vi "Destory for traverse.vi"(8 "error in (no error)":errorcluster caption="错误输入（无错误）", 11 "Class in":refnum<class "PanelRootNode.lvclass"> caption="DNL_LabVIEW Object in") -> (0 "error out":errorcluster caption="错误输出", 3 "Class out":refnum<class "PanelRootNode.lvclass"> caption="DNL_LabVIEW Object out")   [LabVIEW 2013, in "PanelRootNode.lvclass"]
uses:
  PanelRootNode.lvclass
  PanelObject/PanelObject.lvclass
  PanelLinkNode/PanelLinkNode.lvclass/PanelLinkNode.ctl
  PanelLinkNode/PanelLinkNode.lvclass
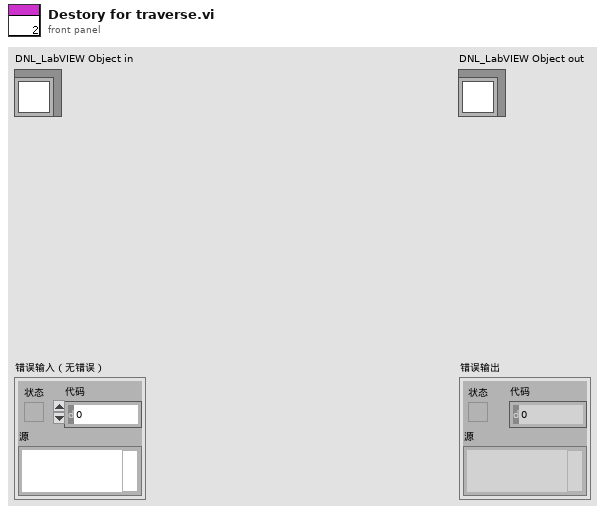
[diagram p1: front panel]
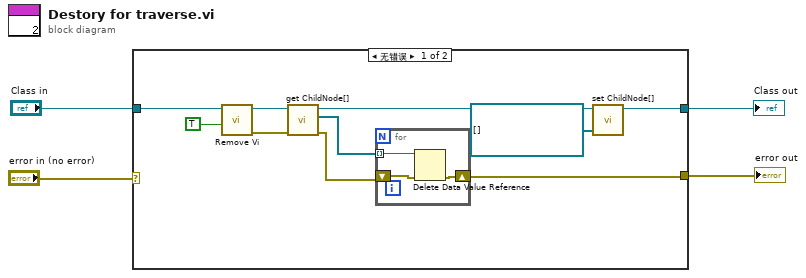
[diagram p0: block diagram]
diagram:
  n1 = case shown="无错误" "error in (no error)" {
    selector: "error in (no error)" -> [_ w19]
    tunnel: [w8 w19] -> w3
    tunnel: [w6 w18] -> w1
    tunnel: "Class in" -> [w13 w18]
    frame No Error {
      n2 = call-dynamic "Remove Vi.vi"("Abort VI"=TRUE, "PanelDataNode 输入"=w13) -> ("error out"=w11:errorcluster, "PanelDataNode 输出"=w12:refnum<class "PanelRootNode.lvclass">)  [unwired: 6 in, 2 out]
      n3 = call "get ChildNode[].vi"("error in (no error)"=w11, "PanelLinkNode输入"=w12) -> ("error out"=w9:errorcluster, "ChildNode*[]"=w10:refnum<data-value>[], "PanelLinkNode输出"=w7:refnum<class "PanelRootNode.lvclass">)  [unwired: 7 in]
      n4 = for {
        tunnel: w10 -> [w17] mode=indexing
        shift-right: [w15] -> w8
        shift-left: w9 -> [w16]
        n5 = Delete Data Value Reference(data value reference=w17, error in=w16) -> (error out=w15:errorcluster)  [unwired: 1 out]
      }
      n6 = call "set ChildNode[].vi"("ChildNode*[]"=refnum<data-value>[] [], "PanelLinkNode输入"=w7) -> ("PanelLinkNode输出"=w6:refnum<class "PanelRootNode.lvclass">)  [unwired: 8 in, 1 out]
    }
    frame Error {
    }
  }
  "error out" <- w3
  "Class out" <- w1
